vi "Prueba Web.vi"(6 "LabVIEW Web Service":refnum<class "Web Service.lvclass">) -> (2 "x*y":dbl)   [LabVIEW 2013]
uses:
  <vilib>/wsapi/Web Service.lvclass
panel:
  # "Use the web service input terminal to call the VIs on the Service subpalette of the Web Services palette. Do not remove it from the connector pane unless you don't need access to the palette."
  # "Any additional terminals added to the connector pane of a startup VI will be ignored."
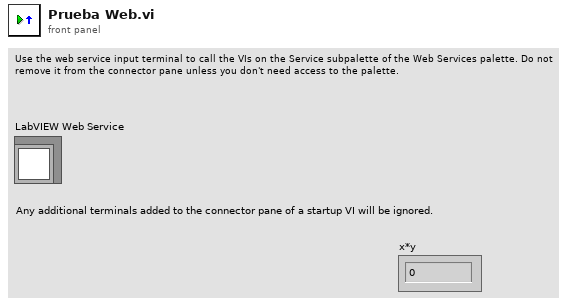
[diagram p1: front panel]
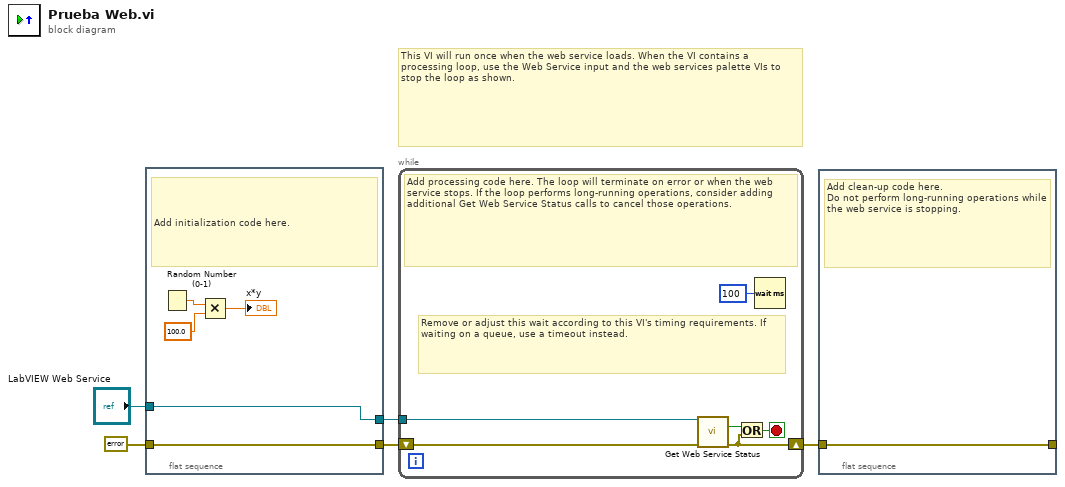
[diagram p0: block diagram]
diagram:
  # "This VI will run once when the web service loads. When the VI contains a processing loop, use the Web Service input and the web services palette VIs to stop the loop as shown."
  n1 = flat-sequence {
    tunnel: "LabVIEW Web Service" -> [w10]
    tunnel: [w10] -> w4
    tunnel: [w9] -> w3
    tunnel: errorcluster {"status"=FALSE, "code"=0, "source"=""} ("error constant") -> [w9]
    frame #0 {
      # "Add initialization code here."
      n2 = Random Number (0-1)() -> (number: 0 to 1=w8:dbl)
      n3 = Multiply(x=w8, y=100.0) -> (x*y=→"x*y":dbl)
    }
  }
  n4 = while {
    tunnel: w4 -> [w15]
    shift-right: [w12] -> w1
    shift-left: w3 -> [w13]
    stop <- w14 stop-if-true
    # "Remove or adjust this wait according to this VI's timing requirements. If waiting on a queue, use a timeout instead."
    # "Add processing code here. The loop will terminate on error or when the web service stops. If the loop performs long-running operations, consider adding additional Get Web Service Status calls to cancel those operations."
    n5 = call <vilib>:"Get Web Service Status.vi"("LabVIEW Web Service"=w15, "error in (no error)"=w13) -> ("service stopping?"=w16:bool, "error out"=w12:errorcluster)  [unwired: 11 in, 1 out]
    n6 = Or(x=w16, y=w12) -> (x .or. y?=w14:bool)
    n7 = Wait (ms)(milliseconds to wait=u32 100) -> ()  [unwired: 1 out]
  }
  n8 = flat-sequence {
    tunnel: [w17] -> _
    tunnel: w1 -> [w17]
    frame #0 {
      # "Add clean-up code here.\nDo not perform long-running operations while the web service is stopping."
    }
  }
